vi "VRM_sweepVsg_lockin.vi"(2 "Comments":string="SA02703M.2014121\n\n Vbg: -5.3V\nsweep Vsg=80mV\nsweep B = 0T to 0.5T to -0.5T to 0T, 0.00214A/s\n\nlockin\n0: 3\n1: 4, bad\n2: 5\n3: 7, current \n4: 9\n5: 2, current 4mV AC, -190uV DC, 400mHz", 3 "ITX folder":string="11 - sweep B", 5 "Sweep rate (A/s)":dbl=0.002, 6 "Measurement type":i32=1, 7 "step size":dbl=0.5 format="%.4f", 8 "Min":dbl=-0.5, 9 "Max":dbl=0.5) -> (0 "error out":errorcluster={"status"=TRUE, "code"=1, "source"="Get Notifier Status in VRM_sweepVsg_lockin.vi"})   [LabVIEW 2013]
uses:
  cryogenic ltd/state machine/state machine/Cryogeni Global 1.vi
  <userlib>/Levylab/DAQ-Lockin-SubVI/Lock-in Globles.vi
panel:
  in  "Rate:\nT=set rate\nF=fastest rate":bool=TRUE
  in  "T=tesla\nF=amps":bool=TRUE
  out "Waveform Graph":dbl[](graph)=[0.0, 0.5, -3.8163916471489756e-17, -0.49999999999999994, 0.0]
  in  "Cryogenic PS":refnum<visa-resource-name>="COM4"
  in  "function (ramp)":enum16{"Ramp", "Triangle", "Sine"}(ring)=enum."Triangle"
  in  "phase":dbl
  in  "cycles (1,2,...)":i32=1 min=1 step=1
  in  "error in (no error)":errorcluster
  in  "stop":bool
  # "0=lockin Vsg\n1=IV\n2=monitor lockin"
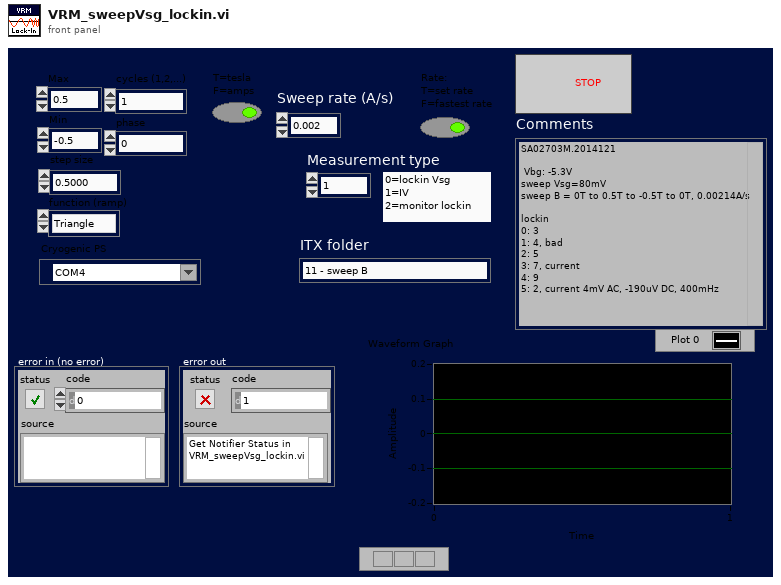
[diagram p1: front panel]
types:
  T1 = cluster{"Ramp Target":enum16{"ZERO", "MID", "MAX"}, "Pause":bool, "Switch Heater":bool, "Persistent Field":dbl, "Persistent Current":dbl, "Tesla":bool, "Output (T)":dbl, "Output (A)":dbl, "X Trip":enum16{"DISABLED", "ENABLED", "ACTIVE"}, "Ramp Rate (A/s)":dbl, "V Limit (V)":dbl, "Heater Voltage":dbl, "MAX Setpoint (A)":dbl, "MAX Setpoint (T)":dbl, "MID Setpoint (A)":dbl, "MID Setpoint (T)":dbl, "Lock":bool, "Field Constant":dbl, "Remote":bool, "Direction":enum16{"POSITIVE", "NEGATIVE", "OPEN", "UNIPOLAR"}, "Helium Level":u16, "Quench !":bool, "Voltage":dbl, "V Limit !":bool, "Ramping":bool, "At Target":bool, "Trip Field":dbl, "Trip Current":dbl}
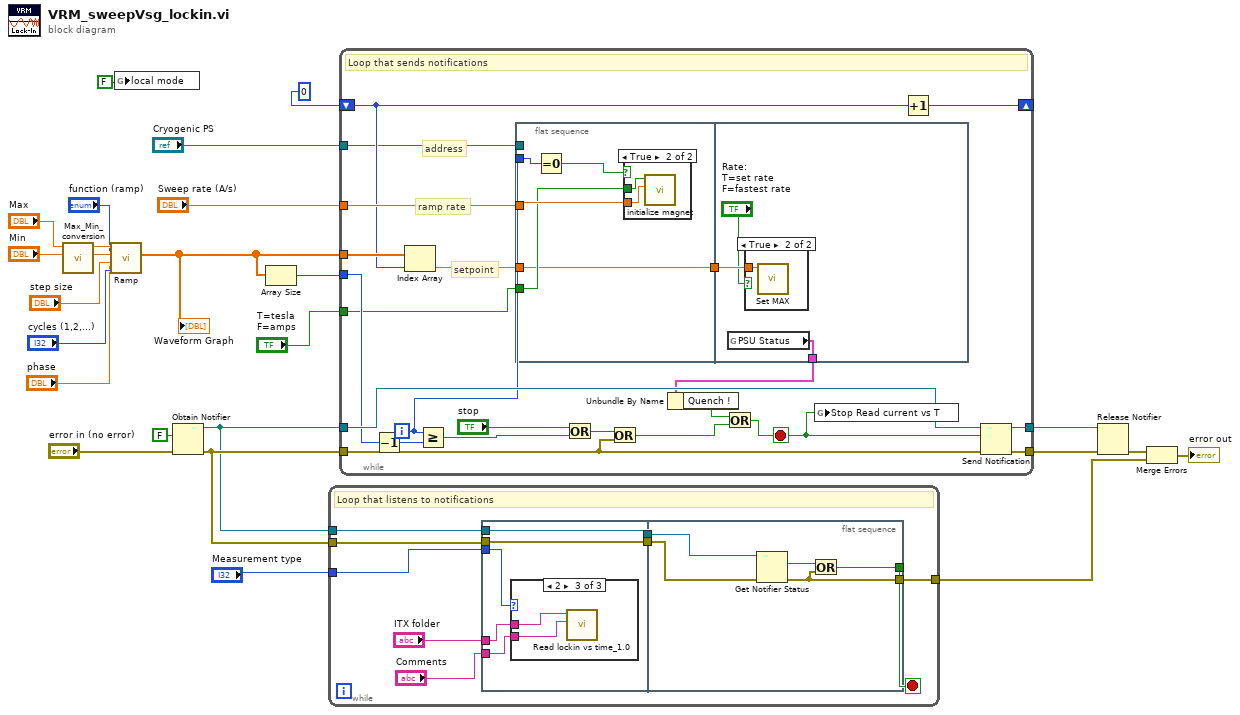
[diagram p0: block diagram]
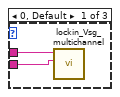
[diagram p2: hidden frame]
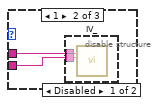
[diagram p3: hidden frame]
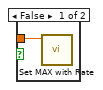
[diagram p6: hidden frame]
diagram:
  n1 = call <userlib>:"Max_Min_conversion.vi"("Min"="Min", "Max"="Max") -> ("offset"=w10:dbl, "Amplitude"=w11:dbl)  [unwired: 8 in]
  n2 = call <userlib>:"Ramp.vi"("phase"="phase", "function (ramp)"="function (ramp)", "cycles (1,2,...)"="cycles (1,2,...)", "step size"="step size", "offset"=w10, "amplitude"=w11) -> ("Waveform Graph"=w4:dbl[])  [unwired: 3 in, 2 out]
  "Waveform Graph" <- w4
  n3 = global write "Cryogeni Global 1.vi" "local mode"(FALSE) -> ()
  n4 = Obtain Notifier(notification data type=FALSE, error in (no error)="error in (no error)") -> (notifier out=w24:refnum<notifier>, error out=w25:errorcluster)  [unwired: 2 in, 1 out]
  n5 = Array Size(array=w4) -> (size(s)=w3:i32)
  n6 = while {
    tunnel: w25 -> [w30]
    tunnel: w24 -> [w32]
    tunnel: "Measurement type" -> [w34]
    tunnel: [w29] -> w14
    stop <- w28 stop-if-true
    # "Loop that listens to notifications"
    n7 = flat-sequence {
      tunnel: w34 -> [w35]
      tunnel: "ITX folder" -> [w39]
      tunnel: "Comments" -> [w38]
      tunnel: [w37] -> w33
      tunnel: w32 -> [w37]
      tunnel: [w36] -> w31
      tunnel: w30 -> [w36]
      tunnel: w33 -> [w52]
      tunnel: w31 -> [w51]
      tunnel: [w50] -> w28
      tunnel: [w49] -> w29
      frame #0 {
        n8 = case shown="2" w35 {
          tunnel: w39 -> [w41 w43 w47]
          tunnel: w38 -> [w40 w42 w46]
          frame 0, Default {
            n9 = call "lockin_Vsg_multichannel.vi"("Comments"=w40, "ITX folder"=w41) -> ()  [unwired: 10 in]
          }
          frame 1 {
            n10 = disable-structure shown="Disabled" {
              disable-tunnel: w43 -> [w45 _]
              disable-tunnel: w42 -> [w44 _]
              frame Disabled {
                n11 = call "IV_.vi"("Notes"=w44, "Experiment folder name"=w45) -> ()  [unwired: 10 in]
              }
              frame Enabled {
              }
            }
          }
          frame 2 {
            n12 = call "Read lockin vs time_1.0.vi"("Comments"=w46, "folder name"=w47) -> ()  [unwired: 7 in, 3 out]
          }
        }
      }
      frame #1 {
        n13 = Get Notifier Status(notifier=w52, error in (no error)=w51) -> (current notification=w48:bool, error out=w49:errorcluster)  [unwired: 3 out]
        n14 = Or(x=w48, y=w49) -> (x .or. y?=w50:bool)
      }
    }
  }
  n15 = while {
    tunnel: w24 -> [w71]
    tunnel: w25 -> [w68]
    tunnel: [w74] -> w15
    tunnel: [w73] -> w23
    tunnel: "Sweep rate (A/s)" -> [w72]
    shift-right: [w66] -> _
    shift-left: 0 -> [w64]
    tunnel: w4 -> [w65]
    tunnel: "Cryogenic PS" -> [w62]
    tunnel: "T=tesla\nF=amps" -> [w61]
    tunnel: w3 -> [w67]
    i -> [w59]
    stop <- w53 stop-if-true
    # "setpoint"
    # "ramp rate"
    # "address"
    # "Loop that sends notifications"
    n16 = Decrement(x=w67) -> (x-1=w56:i32)
    n17 = Index Array(array=w65, index=w64) -> (element=w63:dbl)
    n18 = Greater Or Equal?(x=w59, y=w56) -> (x >= y?=w57:bool)
    n19 = flat-sequence {
      tunnel: w72 -> [w77]
      tunnel: w63 -> [w75]
      tunnel: w62 -> [_]
      tunnel: w61 -> [w76]
      tunnel: w59 -> [w79]
      tunnel: [w75] -> w58
      tunnel: w58 -> [w84]
      tunnel: [w82] -> w55
      frame #0 {
        n20 = Equal To 0?(x=w79) -> (x = 0?=w78:bool)
        n21 = case shown="True" w78 {
          tunnel: w77 -> [_ w81]
          tunnel: w76 -> [_ w80]
          frame False {
          }
          frame True {
            n22 = call "initialize magnet.vi"("Ramp rate (A/s)"=w81, "T=Tesla\nF=Amps"=w80) -> ()  [unwired: 10 in]
          }
        }
      }
      frame #1 {
        n23 = global read "Cryogeni Global 1.vi" "PSU Status"() -> (w82:T1)
        n24 = case shown="True" "Rate:\nT=set rate\nF=fastest rate" {
          tunnel: w84 -> [w85 w86]
          frame False {
            n25 = call "Set MAX with Rate.vi"("setpoint"=w85) -> ()  [unwired: 11 in]
          }
          frame True {
            n26 = call "Set MAX.vi"("setpoint"=w86) -> ()  [unwired: 11 in]
          }
        }
      }
    }
    n27 = Or(x="stop", y=w57) -> (x .or. y?=w69:bool)
    n28 = Or(x=w69, y=w68) -> (x .or. y?=w60:bool)
    n29 = Unbundle By Name(w55) -> ("Quench !"=w54:bool)
    n30 = Or(x=w54, y=w60) -> (x .or. y?=w53:bool)
    n31 = global write "Lock-in Globles.vi" "Stop Read current vs T"(w53) -> ()
    n32 = Increment(x=w64) -> (x+1=w66:i32)
    n33 = Send Notification(notification=w53, notifier=w71, error in (no error)=w68) -> (notifier out=w74:refnum<notifier>, error out=w73:errorcluster)
  }
  n34 = Release Notifier(notifier=w15, error in (no error)=w23) -> (error out=w17:errorcluster)  [unwired: 1 in, 2 out]
  n35 = Merge Errors(w17, w14) -> (→"error out":errorcluster)
